vi "SearchTerminalSourceWire.vi"(8 "error in (no error)":errorcluster, 10 "Source?":bool=TRUE, 11 "Refnum Wire In":refnum<vi>) -> (0 "error out":errorcluster, 2 "Terminal Refnum":refnum<vi>, 3 "Refnum Wire Out":refnum<vi>)   [LabVIEW 2011]
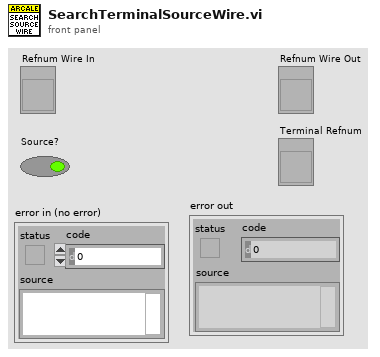
[diagram p1: front panel]
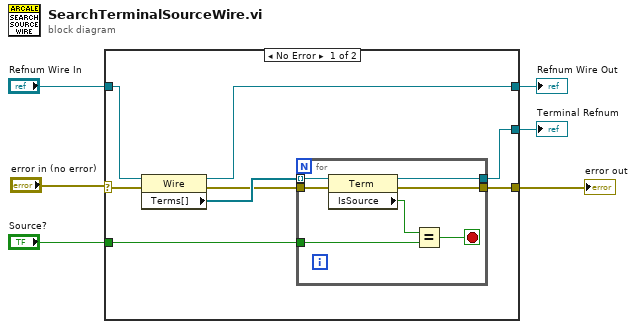
[diagram p0: block diagram]
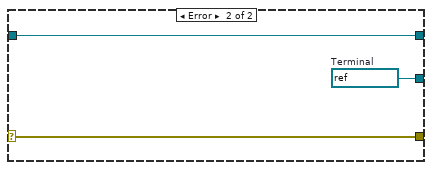
[diagram p2: hidden frame]
diagram:
  n1 = case shown="No Error" "error in (no error)" {
    selector: "error in (no error)" -> [w13 w24]
    tunnel: "Refnum Wire In" -> [w9 w23]
    tunnel: "Source?" -> [w11 _]
    tunnel: [w10 w24] -> w3
    tunnel: [w8 w23] -> w2
    tunnel: [w7 w22] -> w1
    frame No Error {
      n2 = property class="Wire"(reference=w9, error in=w13) -> (reference out=w8:refnum<vi>, error out=w12:errorcluster, "Terms[]"=w14:refnum<vi>[])
      n3 = for {
        tunnel: w14 -> [w21] mode=indexing
        tunnel: [w20] -> w7
        tunnel: w12 -> [w19]
        tunnel: [w18] -> w10
        tunnel: w11 -> [w16]
        stop <- w15 stop-if-true
        n4 = property class="Term"(reference=w21, error in=w19) -> (reference out=w20:refnum<vi>, error out=w18:errorcluster, "IsSource"=w17:bool)
        n5 = Equal?(x=w17, y=w16) -> (x = y?=w15:bool)
      }
    }
    frame Error {
      w22 = refnum<vi> refnum  # Terminal
    }
  }
  "error out" <- w3
  "Refnum Wire Out" <- w2
  "Terminal Refnum" <- w1
